vi "Map to Array.vi"(11 "map":map{string, dbl}(c390)) -> (2 "States":dbl[](array[numeric]), 3 "Keys":string[](array[string]))   [LabVIEW 2024, in "Logger.lvlib"]
uses:
  Logger.lvlib
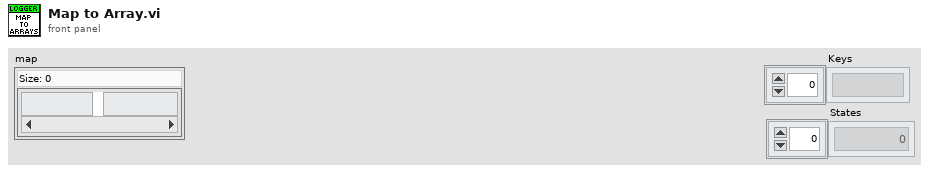
[diagram p1: front panel]
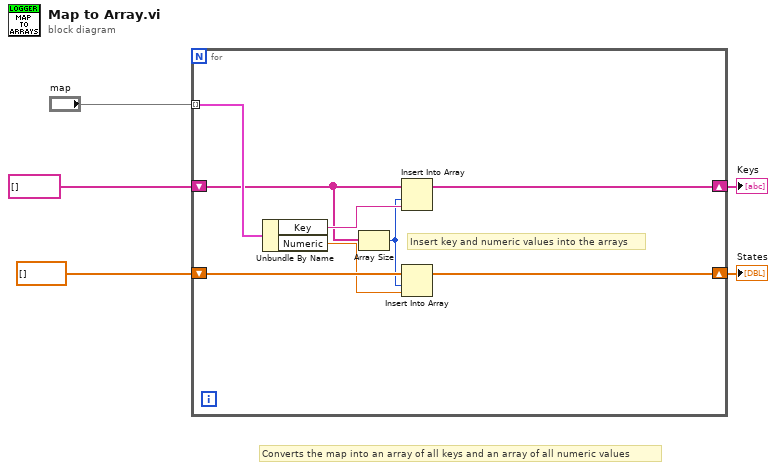
[diagram p0: block diagram]
diagram:
  # "Converts the map into an array of all keys and an array of all numeric values"
  n1 = for {
    tunnel: "map" -> [w12] mode=indexing
    shift-right: [w13] -> w2
    shift-left: string[] [] -> [w7]
    shift-right: [w9] -> w1
    shift-left: dbl[] [] -> [w10]
    # "Insert key and numeric values into the arrays"
    n2 = Unbundle By Name(w12) -> ("Key"=w11:string, "Numeric"=w8:dbl)
    n3 = Array Size(array=w7) -> (size(s)=w6:i32)
    n4 = Insert Into Array(array=w7, index=w6, new element=w11) -> (w13:string[])
    n5 = Insert Into Array(array=w10, index=w6, new element=w8) -> (w9:dbl[])
  }
  "Keys" <- w2
  "States" <- w1
